vi "探头模块-精简版-35点.vi"() -> ()   [LabVIEW 2013]
panel:
  in  "报警状态？":refnum<vi>
  in  "数组":bool[](array[boolean])
  in  "测量值":refnum<vi>
  in  "更新列表？":refnum<vi>
  in  "引用传入":T1
  out "停止":bool=TRUE
  in  "探头启用状态？":refnum<vi>
  in  "更新显示？":bool
  in  "备注信息":refnum<vi>
  out "探头 35":T3
  out "探头 34":T3
  out "探头 33":T3
  out "探头 32":T3
  out "探头 31":T3
  out "探头 30":T3
  out "探头 29":T3
  out "探头 28":T3
  out "探头 27":T3
  out "探头 26":T3
  out "探头 25":T3
  out "探头 24":T3
  out "探头 23":T3
  out "探头 22":T3
  out "探头 21":T3
  out "探头 20":T3
  out "探头 19":T3
  out "探头 18":T3
  out "探头 17":T3
  out "探头 16":T3
  out "探头 15":T3
  out "探头 14":T3
  out "探头 13":T3
  out "探头 12":T3
  out "探头 11":T3
  out "探头 10":T3
  out "探头 9":T3
  out "探头 8":T3
  out "探头 7":T3
  out "探头 6":T3
  out "探头 5":T3
  out "探头 4":T3
  out "探头 3":T3
  out "探头 2":T3
  out "探头 1":T3
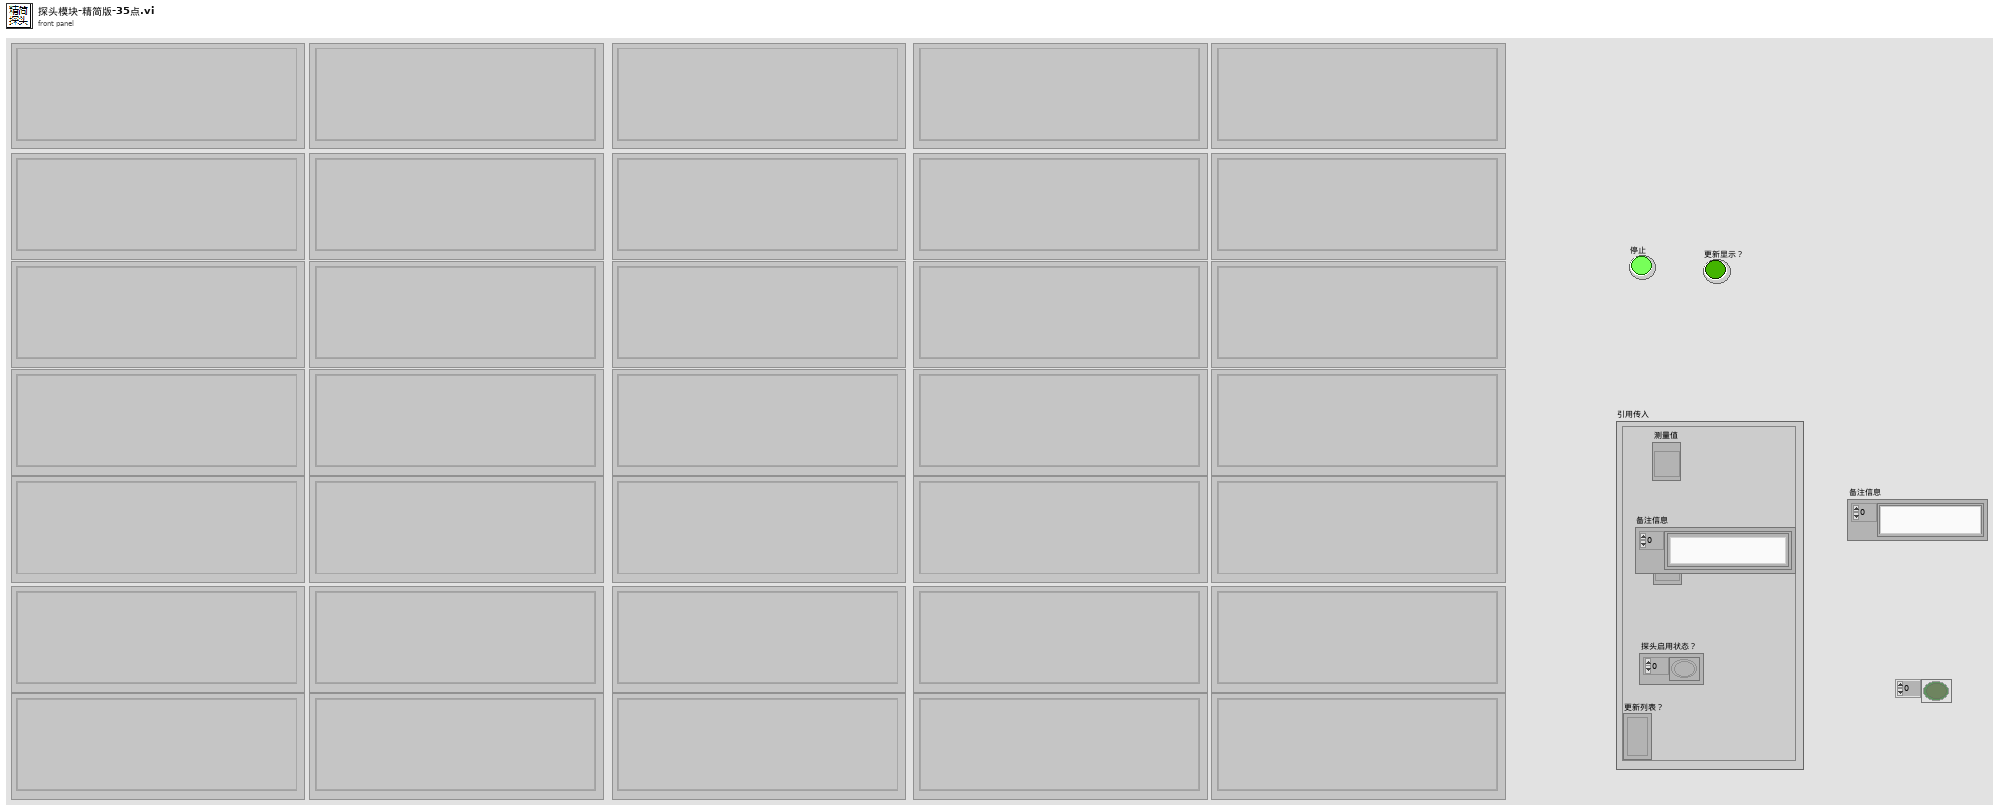
[diagram p1: front panel]
types:
  T1 = cluster{"测量值":refnum<vi>, "备注信息":refnum<vi>, "报警状态？":refnum<vi>, "探头启用状态？":refnum<vi>, "更新列表？":refnum<vi>}
  T2 = typedef "精简探头背景按键.ctl" = bool
  T3 = cluster{"单位":string, "备注信息":string, "测量值":string, "背景":T2}
  T4 = enum8{"Enabled", "Disabled", "Disabled and Grayed Out"}
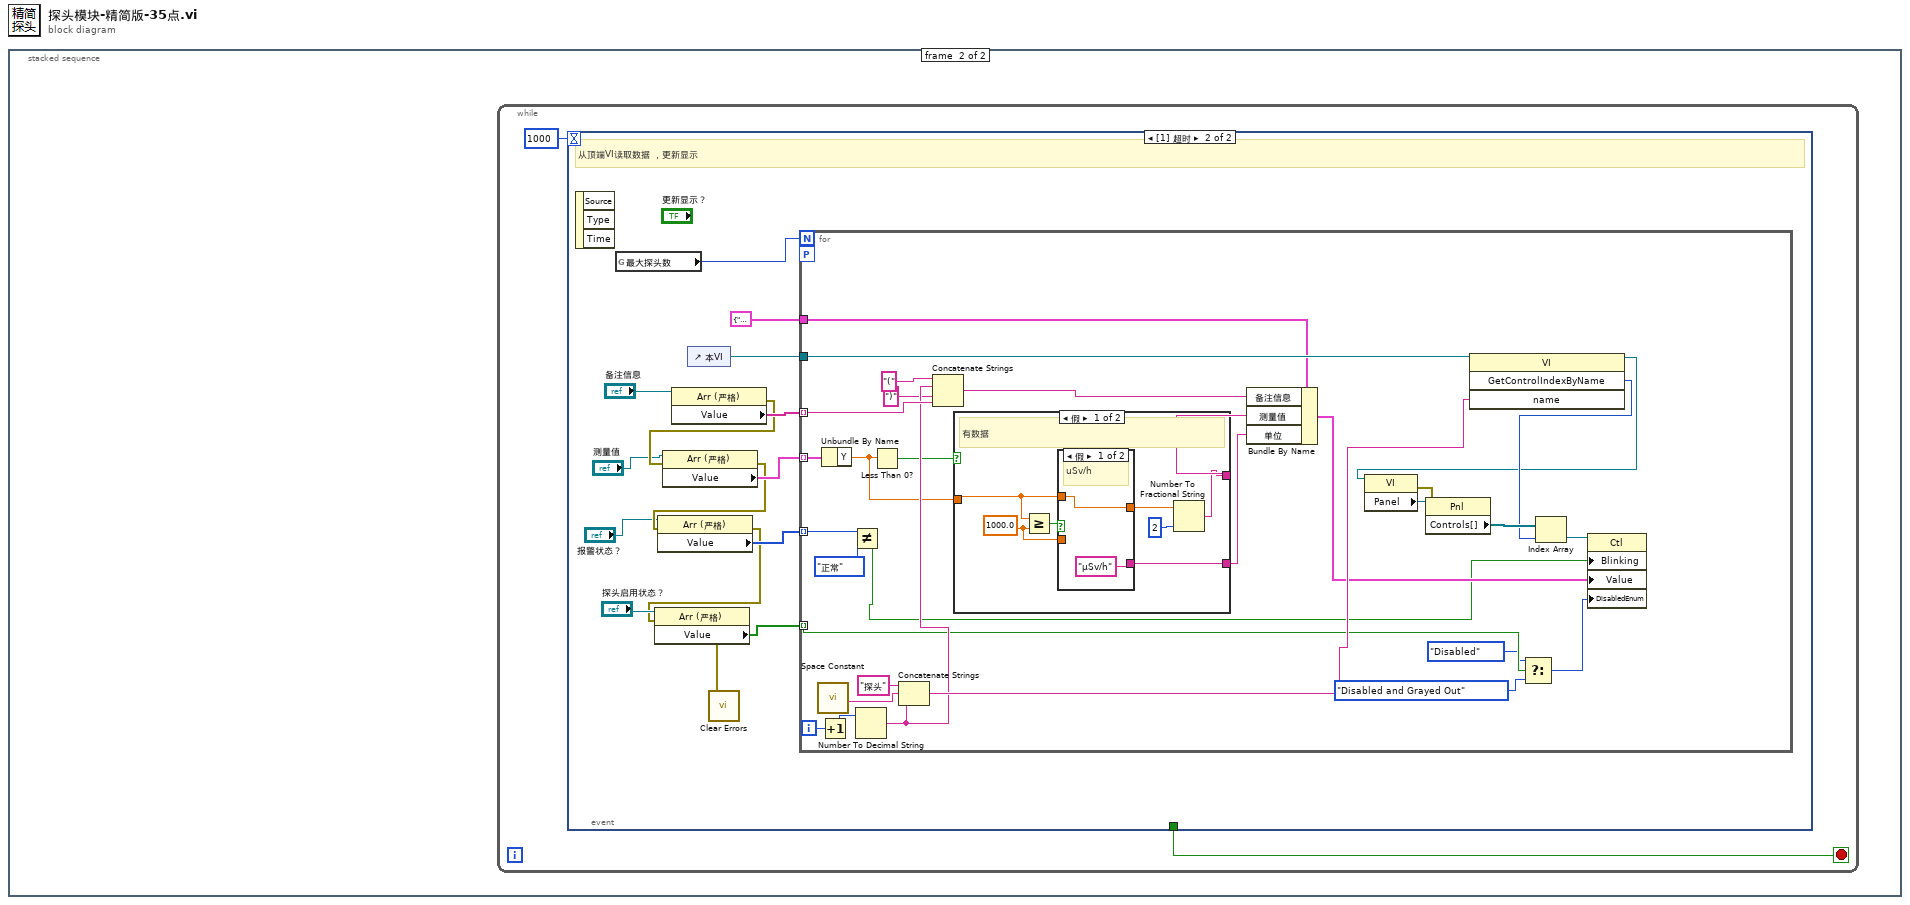
[diagram p0: block diagram]
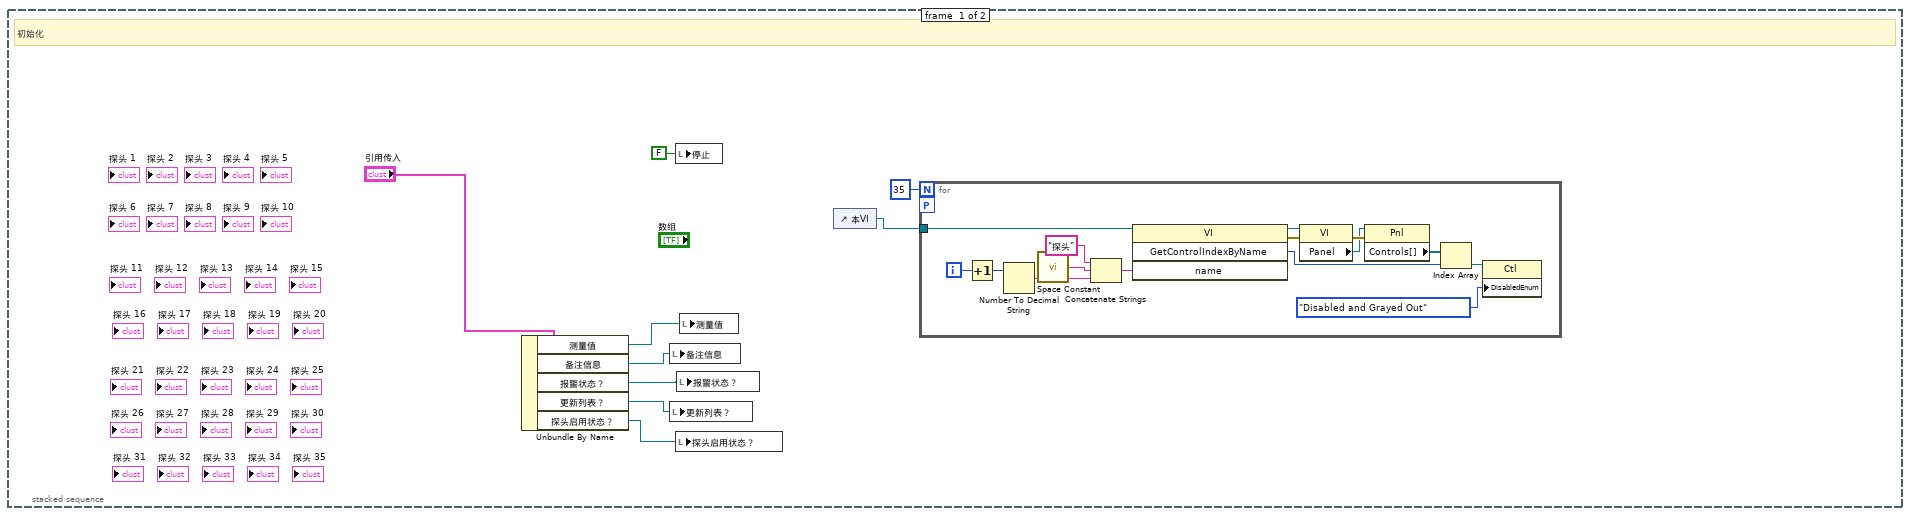
[diagram p2: hidden frame]
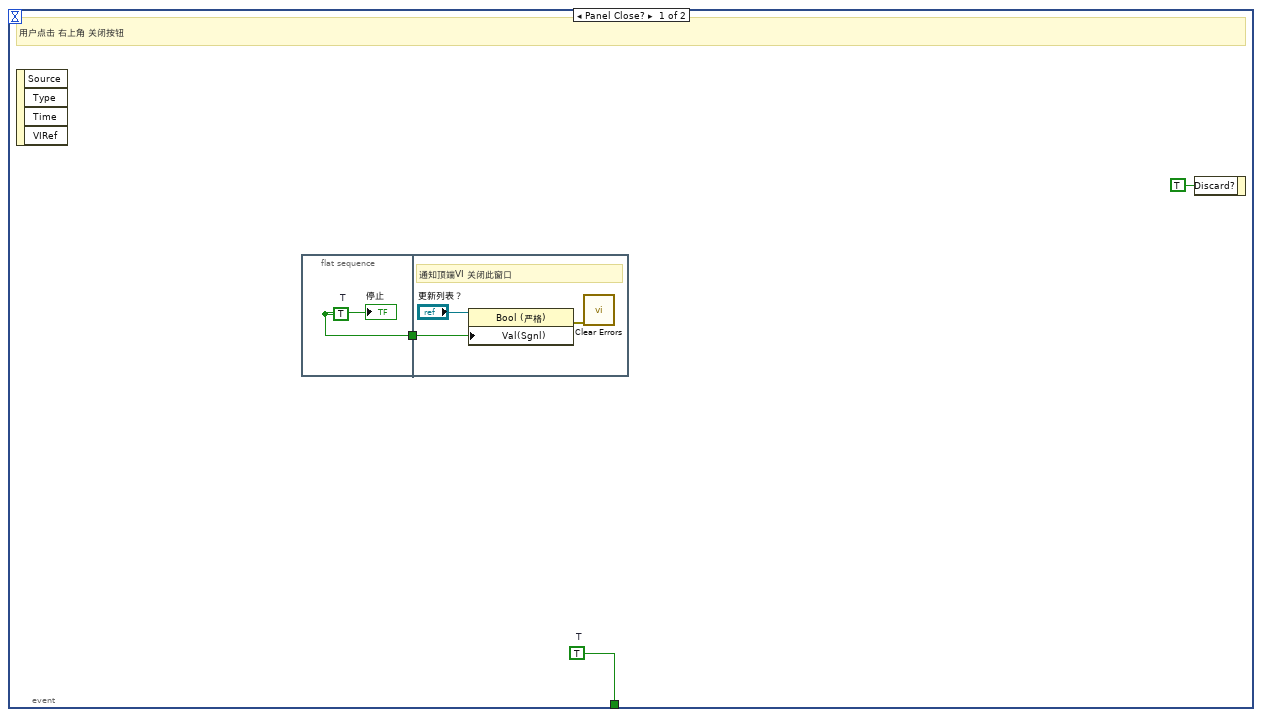
[diagram p3: hidden frame]
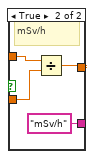
[diagram p4: hidden frame]
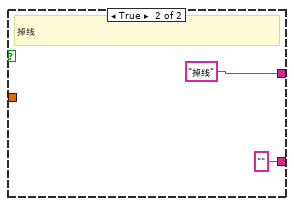
[diagram p5: hidden frame]
diagram:
  n1 = stacked-sequence {
    frame #0 {
      # "初始化"
      n2 = Unbundle By Name("引用传入") -> ("测量值"=w2:refnum<vi>, "备注信息"=w7:refnum<vi>, "报警状态？"=w1:refnum<vi>, "更新列表？"=w5:refnum<vi>, "探头启用状态？"=w8:refnum<vi>)
      n3 = local write "备注信息"(w7) -> ()
      n4 = local write "更新列表？"(w5) -> ()
      n5 = local write "停止"(FALSE ("停止")) -> ()
      n6 = local write "探头启用状态？"(w8) -> ()
      n7 = local write "报警状态？"(w1) -> ()
      n8 = local write "测量值"(w2) -> ()
      n9 = control-ref of="本VI"() -> (w4:refnum<vi>)
      n10 = for {
        N: 35 -> [_]
        tunnel: w4 -> [w24]
        workers-P: _ -> [_]
        i -> [w19]
        n11 = Increment(x=w19) -> (x+1=w21:i32)
        n12 = Number To Decimal String(number=w21) -> (decimal integer string=w20:string)  [unwired: 1 in]
        n13 = call <vilib>:"Space Constant.vi"() -> ("String"=w22:string)
        n14 = Concatenate Strings("探头" ("字符串"), w22, w20) -> (w18:string)
        n15 = invoke class="VI" method="GetControlIndexByName"(reference=w24, "name"=w18) -> (reference out=w17:refnum<vi>, error out=w16:errorcluster, "GetControlIndexByName"=w12:i32)  [unwired: 2 in, 1 out]
        n16 = property class="VI"(reference=w17, error in=w16) -> (error out=w15:errorcluster, "Panel"=w14:refnum<vi>)  [unwired: 1 out]
        n17 = property class="Pnl"(reference=w14, error in=w15) -> ("Controls[]"=w13:refnum<vi>[])  [unwired: 2 out]
        n18 = Index Array(array=w13, index=w12) -> (element=w11:refnum<vi>)
        n19 = property class="Ctl"(reference=w11, "DisabledEnum"=T4."Disabled and Grayed Out" ("禁用")) -> ()  [unwired: 1 in, 2 out]
      }
    }
    frame #1 {
      n20 = while {
        stop <- w26 stop-if-true
        n21 = event shown="[1] 超时" {
          selector: _ -> [_ _]
          dyn-events: _ -> [_ _]
          timeout: 1000 -> [_ _]
          tunnel: [w28 _] -> w26
          event Panel Close? {
            w28 = TRUE  # T
            # "用户点击 右上角 关闭按钮"
            n22 = event-data() -> ()  [unwired: 1 in, 4 out]
            n23 = flat-sequence {
              tunnel: [w30] -> w27
              tunnel: w27 -> [w32]
              frame #0 {
                w30 = TRUE  # T
                "停止" <- w30
              }
              frame #1 {
                # "通知顶端VI 关闭此窗口"
                n24 = property class="Bool (严格)"(reference="更新列表？", "Val(Sgnl)"=w32) -> (error out=w31:errorcluster)  [unwired: 1 in, 1 out]
                n25 = call <vilib>:"Clear Errors.vi"("error in (no error)"=w31) -> ()  [unwired: 6 in, 1 out]
              }
            }
            n26 = event-data("Discard?"=TRUE ("放弃？")) -> ()  [unwired: 1 in, 1 out]
          }
          event Timeout {
            # "从顶端VI读取数据 ，更新显示"
            n27 = event-data() -> ()  [unwired: 1 in, 3 out]
            n28 = global read "全局变量-35点监测.vi" "最大探头数"() -> (w40:i32)
            n29 = property class="Arr (严格)"(reference="备注信息") -> (error out=w39:errorcluster, "Value"=w45:string[])  [unwired: 1 in, 1 out]
            n30 = property class="Arr (严格)"(reference="测量值", error in=w39) -> (error out=w38:errorcluster, "Value"=w44:cluster{"X":timestamp, "Y":dbl}[])  [unwired: 1 out]
            n31 = property class="Arr (严格)"(reference="报警状态？", error in=w38) -> (error out=w37:errorcluster, "Value"=w42:enum16{"正常", "一级报警", "二级报警"}[])  [unwired: 1 out]
            n32 = property class="Arr (严格)"(reference="探头启用状态？", error in=w37) -> (error out=w36:errorcluster, "Value"=w41:bool[])  [unwired: 1 out]
            n33 = control-ref of="本VI"() -> (w48:refnum<vi>)
            n34 = call <vilib>:"Clear Errors.vi"("error in (no error)"=w36) -> ()  [unwired: 6 in, 1 out]
            n35 = for {
              N: w40 -> [_]
              tunnel: w48 -> [w79]
              workers-P: _ -> [_]
              tunnel: T3 {"单位"="mSv/h", "备注信息"="4号楼509-邢均儒", "测量值"="0.15", "背景"=TRUE} ("探头 25") -> [w78]
              tunnel: w45 -> [w73] mode=indexing
              tunnel: w44 -> [w70] mode=indexing
              tunnel: w42 -> [w69] mode=indexing
              tunnel: w41 -> [w55] mode=indexing
              i -> [w75]
              n36 = call <vilib>:"Space Constant.vi"() -> ("String"=w76:string)
              n37 = Increment(x=w75) -> (x+1=w72:i32)
              n38 = Unbundle By Name(w70) -> ("Y"=w51:dbl)
              n39 = Not Equal?(x=w69, y=enum16{"正常", "一级报警", "二级报警"}."正常") -> (x != y?=w50:bool)
              n40 = Number To Decimal String(number=w72) -> (decimal integer string=w71:string)  [unwired: 1 in]
              n41 = Less Than 0?(x=w51) -> (x < 0?=w56:bool)
              n42 = Concatenate Strings("探头" ("字符串"), w76, w71) -> (w74:string)
              n43 = Concatenate Strings("(" ("字符串"), w71, ")" ("字符串"), w73) -> (w66:string)
              n44 = case shown="假" w56 {
                tunnel: [w81 "掉线" ("字符串")] -> w65
                tunnel: w51 -> [w86 _]
                tunnel: [w80 "" ("字符串")] -> w64
                frame False {
                  w84 = 1000.0 ("y")
                  # "有数据"
                  n45 = Greater Or Equal?(x=w86, y=w84) -> (x >= y?=w85:bool)
                  n46 = case shown="假" w85 {
                    tunnel: w86 -> [w88 w92]
                    tunnel: w84 -> [_ w91]
                    tunnel: [w88 w90] -> w82
                    tunnel: ["μSv/h" ("字符串") "mSv/h" ("字符串")] -> w80
                    frame False {
                      # "uSv/h"
                    }
                    frame True {
                      # "mSv/h"
                      n47 = Divide(x=w92, y=w91) -> (x/y=w90:dbl)
                    }
                  }
                  n48 = Number To Fractional String(number=w82, precision (6)=i16 2 ("精度(6)")) -> (F-format string=w81:string)  [unwired: 2 in]
                }
                frame True {
                  # "掉线"
                }
              }
              n49 = Bundle By Name(cluster=w78, "备注信息"=w66, "测量值"=w65, "单位"=w64) -> (w57:T3)
              n50 = invoke class="VI" method="GetControlIndexByName"(reference=w79, "name"=w74) -> (reference out=w58:refnum<vi>, "GetControlIndexByName"=w60:i32)  [unwired: 2 in, 2 out]
              n51 = property class="VI"(reference=w58) -> (error out=w63:errorcluster, "Panel"=w62:refnum<vi>)  [unwired: 1 in, 1 out]
              n52 = property class="Pnl"(reference=w62, error in=w63) -> ("Controls[]"=w61:refnum<vi>[])  [unwired: 2 out]
              n53 = Select(t=T4."Disabled" ("禁用"), s=w55, f=T4."Disabled and Grayed Out" ("禁用")) -> (s? t:f=w52:T4)
              n54 = Index Array(array=w61, index=w60) -> (element=w59:refnum<vi>)
              n55 = property class="Ctl"(reference=w59, "Blinking"=w50, "Value"=w57, "DisabledEnum"=w52) -> ()  [unwired: 1 in, 2 out]
            }
          }
        }
      }
    }
  }
